vi "Get StationGlobals.vi"(8 "error in (no error)":errorcluster, 11 "Session Handle in":T2) -> (0 "error out":errorcluster, 2 "StationGlobals":T1, 3 "Session Handle out":T2)   [LabVIEW 2020, in "HTS.lvlib" / "Engine.lvclass"]
uses:
  Engine/Engine.lvclass
  Engine/Typedefs/Session Handle.ctl
  Typedefs/Session Handle.ctl
  VariableContainer.lvclass
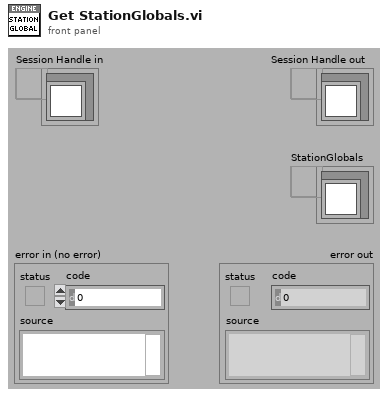
[diagram p1: front panel]
types:
  T1 = typedef "HTS.lvlib/VariableContainer.lvclass/Session Handle.ctl" = refnum<data-value>
  T2 = typedef "HTS.lvlib/Engine.lvclass/Session Handle.ctl" = refnum<data-value>
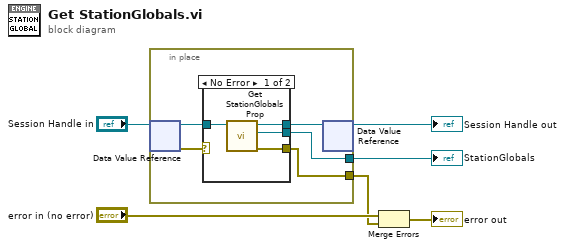
[diagram p0: block diagram]
diagram:
  n1 = in-place {
    in-place-border: [w8] -> w2
    in-place-border: [w7] -> w1
    n2 = in-place-dvr #1("Session Handle in") -> (w11:refnum<class "Engine.lvclass">, w9:errorcluster)
    n3 = case shown="No Error" w9 {
      selector: w9 -> [_ w17]
      tunnel: w11 -> [w15 w16]
      tunnel: [w14 w16] -> w10
      tunnel: [w13 w17] -> w8
      tunnel: [w12 _] -> w7
      frame No Error {
        n4 = call "Get StationGlobals Prop.vi"("TSEngine in"=w15) -> ("error out"=w13:errorcluster, "StationGlobals"=w12:T1, "TSEngine out"=w14:refnum<class "Engine.lvclass">)  [unwired: 8 in]
      }
      frame Error {
      }
    }
    n5 = in-place-dvr #1(w10) -> (→"Session Handle out":T2)  [unwired: 1 out]
  }
  "StationGlobals" <- w1
  n6 = Merge Errors("error in (no error)", w2) -> (→"error out":errorcluster)
